vi "__SR530_init.vi"(7 "GPIB":string="29") -> ()   [LabVIEW 2017]
panel:
  out "l 2":dbl=0.0027
  out "l":dbl=18.0
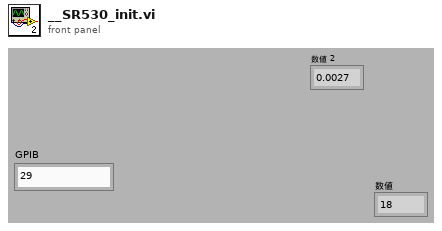
[diagram p1: front panel]
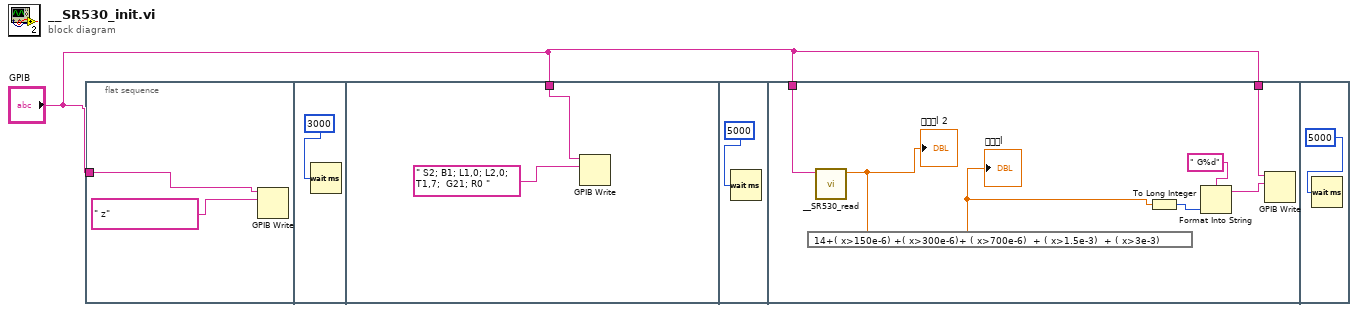
[diagram p0: block diagram]
diagram:
  n1 = flat-sequence {
    tunnel: "GPIB" -> [w3]
    tunnel: "GPIB" -> [w5]
    tunnel: "GPIB" -> [w14]
    tunnel: "GPIB" -> [w8]
    frame #0 {
      n2 = GPIB Write(0:w3, 1:" z") -> ()  [unwired: 3 in, 2 out]
    }
    frame #1 {
      n3 = Wait (ms)(milliseconds to wait=3000) -> ()  [unwired: 1 out]
    }
    frame #2 {
      n4 = GPIB Write(0:w5, 1:" S2; B1; L1,0; L2,0; T1,7;  G21; R0 ") -> ()  [unwired: 3 in, 2 out]
    }
    frame #3 {
      n5 = Wait (ms)(milliseconds to wait=5000) -> ()  [unwired: 1 out]
    }
    frame #4 {
      n6 = call "__SR530_read.vi"("GPIB"=w14) -> ("R"=w13:dbl)  [unwired: 5 in, 1 out]
      "l 2" <- w13
      n7 = expression code="14+( x>150e-6) +( x>300e-6)+ ( x>700e-6)  + ( x>1.5e-3)  + ( x>3e-3)"(w13) -> (w12:dbl)
      "l" <- w12
      n8 = To Long Integer(number=w12) -> (32bit integer=w10:i32)
      n9 = Format Into String(format string=" G%d", w10) -> (resulting string=w9:string)  [unwired: 2 in, 1 out]
      n10 = GPIB Write(0:w8, 1:w9) -> ()  [unwired: 3 in, 2 out]
    }
    frame #5 {
      n11 = Wait (ms)(milliseconds to wait=5000) -> ()  [unwired: 1 out]
    }
  }
